vi "_PC_Daemon_MSConf_SetCommunication.vi"(8 "error in (no error)":errorcluster, 11 "Communication.Param":T1) -> (0 "error out":errorcluster)   [LabVIEW 2018]
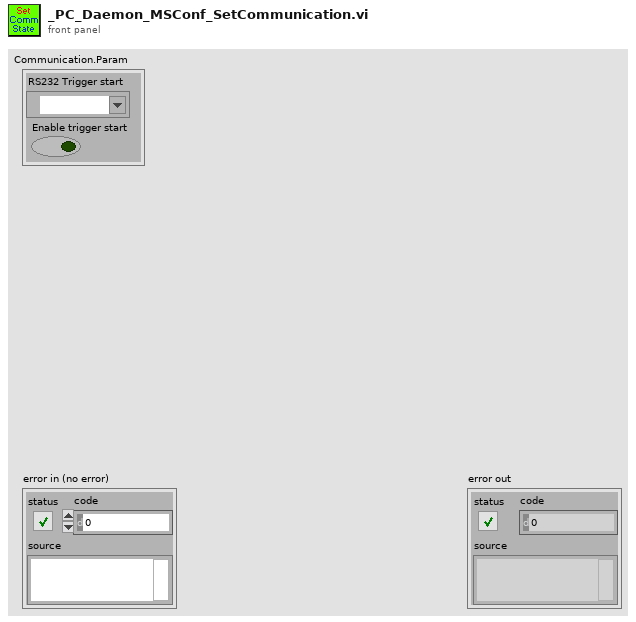
[diagram p1: front panel]
types:
  T1 = cluster{"RS232 Trigger start":refnum<visa-resource-name>, "Enable trigger start":bool}
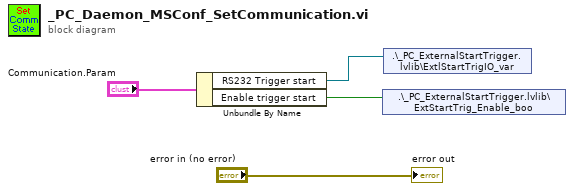
[diagram p0: block diagram]
diagram:
  n1 = Unbundle By Name("Communication.Param") -> ("RS232 Trigger start"=w3:refnum<visa-resource-name>, "Enable trigger start"=w2:bool)
  n2 = shared-variable ".\\_PC_ExternalStartTrigger.lvlib\\ExtStartTrig_Enable_boo"(w2) -> ()  [unwired: 1 in, 1 out]
  n3 = shared-variable ".\\_PC_ExternalStartTrigger.lvlib\\ExtlStartTrigIO_var"(w3) -> ()  [unwired: 1 in, 1 out]
  "error out" <- "error in (no error)"
